vi "Display Console View.vi"(8 "error in (no error)":errorcluster, 11 "View Model":T1) -> (0 "error out":errorcluster, 3 "View Model":T1)   [LabVIEW 2017]
doc: "The interface where user receives status updates from the ATM Controller.\n[Covers: UI3]"
uses:
  View Model/Controls/View Model.ctl
  Error Handler/Controls/Error Model.ctl
  Error Handler/Controls/Error Data.ctl
  Error Handler/Controls/Error Type.ctl
  View Model/Controls/Shared Model.ctl
  Configuration/Controls/Config Model.ctl
  Configuration/Controls/Config CMD.ctl
  Configuration/Controls/Config Data.ctl
  ATM Controller/Controls/Controller Model.ctl
  ATM Controller/Controls/Controller Overhead.ctl
  ATM Controller/Controls/Controller States.ctl
  Controls/Display Console - Message Data.ctl
  Controls/Display Console - Message Name.ctl
  User Console View/Controls/User Console - Keypad.ctl
  User Console View/Controls/User Console - Transactions.ctl
  ATM Controller/Controls/Controller CMD.ctl
panel:
  out "Card Read":bool
  out "Message Screen":string
  out "Current Transaction":string
  # "[Covers: UI3B]"
  # "[Covers: UI3C]"
  # "[Covers: UI3A]"
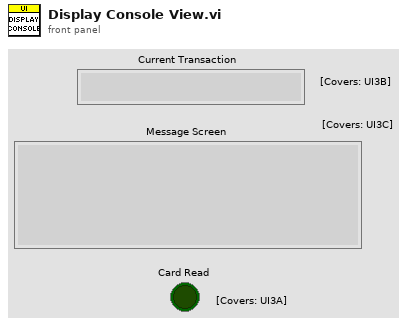
[diagram p1: front panel]
types:
  T1 = typedef "View Model.ctl" = cluster{"Error Model":T2, "Shared Model":T3, "Config Model":T4, "Controller Model":T5}
  T2 = typedef "Error Model.ctl" = cluster{"Error Event":refnum<user-event>}
  T3 = typedef "Shared Model.ctl" = cluster{"Stop Event":refnum<user-event>, "Stop DVR":refnum<data-value>}
  T4 = typedef "Config Model.ctl" = cluster{"Config CMD":refnum<user-event>, "Config Data DVR":refnum<data-value>}
  T5 = typedef "Controller Model.ctl" = cluster{"Controller Overhead DVR":refnum<data-value>, "Deposit Received Change":refnum<user-event>, "Fund Transaction Change":refnum<user-event>, "Card Read Change":refnum<user-event>, "Keypad Change":refnum<user-event>, "Transaction Change":refnum<user-event>, "Controller CMD Change":refnum<user-event>}
  T6 = typedef "Display Console - Message Name.ctl" = enum16{"Welcome", "Idle", "Invalid Login", "Terminate", "Deposit", "Withdrawal", "Fast Cash", "Withdrawal Complete", "Withdrawal Failed", "Balance Inquiry"}
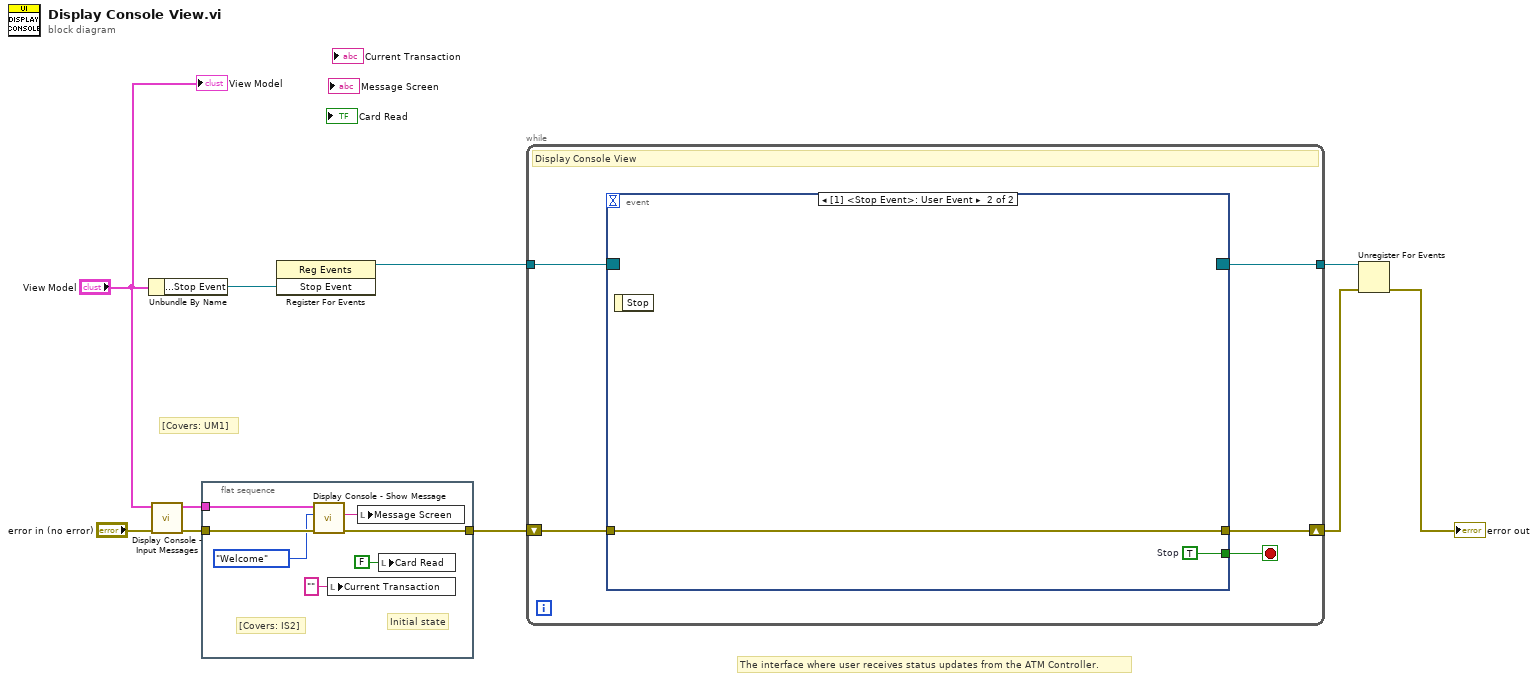
[diagram p0: block diagram]
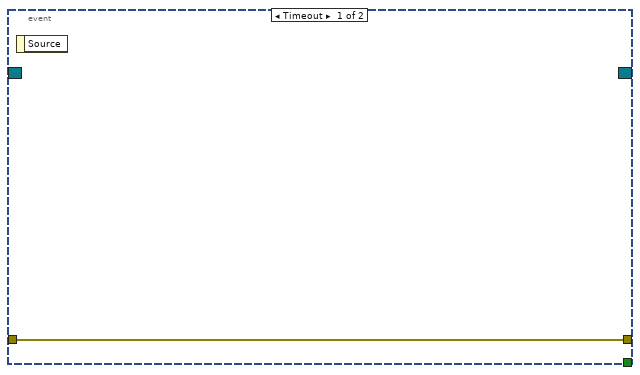
[diagram p2: hidden frame]
diagram:
  # "[Covers: UM1]"
  # "The interface where user receives status updates from the ATM Controller."
  n1 = Unbundle By Name("View Model") -> ("Shared Model.Stop Event"=w10:refnum<user-event>)
  n2 = call "Display Console - Input Messages.vi"("error in (no error)"="error in (no error)", "View Model"="View Model") -> ("error out"=w2:errorcluster, "View Model"=w1:T1)  [unwired: 8 in]
  n3 = flat-sequence {
    tunnel: w2 -> [w14]
    tunnel: [w13] -> w5
    tunnel: w1 -> [w15]
    frame #0 {
      # "[Covers: IS2]"
      # "Initial state"
      n4 = call "Display Console - Show Message.vi"("error in (no error)"=w14, "Message Name"=Display_Console_-_Message_Name."Welcome", "View Model"=w15) -> ("error out"=w13:errorcluster, "Message"=w12:string)  [unwired: 7 in]
      n5 = local write "Current Transaction"("" ("Current Transaction")) -> ()
      n6 = local write "Message Screen"(w12) -> ()
      n7 = local write "Card Read"(FALSE ("Card Read")) -> ()
    }
  }
  n8 = register-events(w10) -> (reference out=w9:refnum<event-registration>)  [unwired: 2 in, 1 out]
  n9 = while {
    tunnel: w9 -> [w22]
    shift-right: [w19] -> w7
    shift-left: w5 -> [w20]
    tunnel: [w18] -> w8
    stop <- w21 stop-if-true
    # "Display Console View"
    n10 = event shown="[1] <Stop Event>: User Event" {
      selector: w22 -> [_ _]
      dyn-events: [_ _] -> w18
      timeout: _ -> [_ _]
      tunnel: [_ w25] -> w21
      tunnel: w20 -> [w23 w24]
      tunnel: [w23 w24] -> w19
      event Timeout {
        n11 = event-data() -> ()  [unwired: 1 in, 1 out]
      }
      event User Event {
        w25 = TRUE  # Stop
        n12 = event-data() -> ()  [unwired: 1 in, 1 out]
      }
    }
  }
  n13 = Unregister For Events(event registration refnum=w8, error in=w7) -> (error out=→"error out":errorcluster)
  "View Model" <- "View Model"
